vi "to_json.vi"(8 "error in":errorcluster, 11 "video in":refnum<class "video.lvclass">) -> (0 "error out":errorcluster, 2 "json":string, 3 "video out":refnum<class "video.lvclass">, 4 "Not Default":bool)   [LabVIEW 2020, in "datasources.lvlib" / "video.lvclass"]
uses:
  video.lvclass
  video.lvclass/video.ctl
  <vilib>/JDP Science/JSONtext/JSONtext.lvlib
  nominal types/timestampManifest/timestampManifest/timestampManifest.lvclass
  target/target.lvclass
  source/source.lvclass
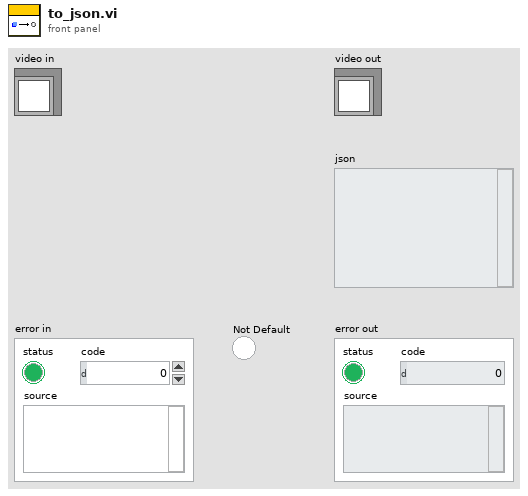
[diagram p1: front panel]
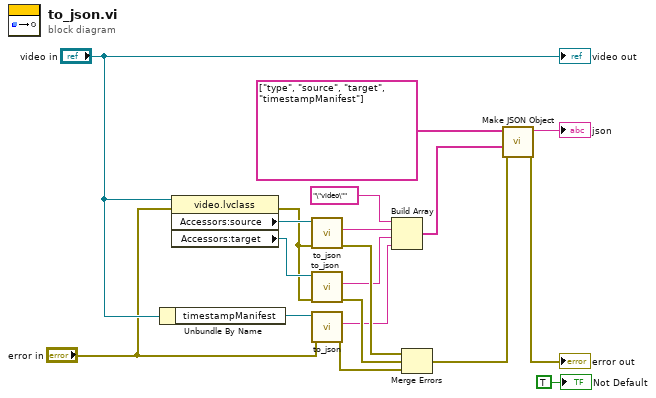
[diagram p0: block diagram]
diagram:
  n1 = Unbundle By Name("video in") -> ("timestampManifest"=w12:refnum<class "timestampManifest.lvclass">)
  n2 = property class="video.lvclass"(reference="video in", error in="error in") -> (error out=w10:errorcluster, "Accessors:source"=w19:refnum<class "source.lvclass">, "Accessors:target"=w18:refnum<class "target.lvclass">)  [unwired: 1 out]
  n3 = call-dynamic "to_json.vi"("error in"=w10, "source in"=w19) -> ("error out"=w8:errorcluster, "json"=w16:string)  [unwired: 6 in, 2 out]
  n4 = call-dynamic "to_json.vi"("error in"=w10, "target in"=w18) -> ("error out"=w7:errorcluster, "json"=w3:string)  [unwired: 6 in, 2 out]
  n5 = call-dynamic "to_json.vi"("error in"="error in", "timestampManifest in"=w12) -> ("error out"=w6:errorcluster, "json"=w2:string)  [unwired: 6 in, 2 out]
  n6 = Build Array("\"video\"" ("element"), w16, w3, w2) -> (w14:string[])
  n7 = Merge Errors(w8, w7, w6) -> (w5:errorcluster)
  n8 = call <vilib>:"Make JSON Object.vi"("error in (no error)"=w5, "JSON Items"=w14, "Item Names"=string[] ["type", "source", "target", "timestampManifest"]) -> ("error out"=→"error out":errorcluster, "<JSON>"=→"json":string)  [unwired: 7 in]
  "video out" <- "video in"
  "Not Default" <- TRUE ("Not Default")
